vi "Thermal Chamber Response Simulator_Init-setup.vi"(11 "test case ID":string) -> (3 "Test Error":errorcluster)   [LabVIEW 2018]
doc: "The setup VI should be executed before the VI under test in the harness VI. In this VI you can prepare the environment and the inputs of the VI under test.\n\nSee the Help Document for more information. (<b>Help</b> > <b>IncQuery Labs</b> > <b>InstaCoverage</b> > <b>InstaCoverage Help...</b>)"
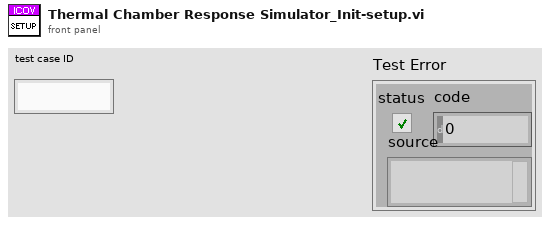
[diagram p1: front panel]
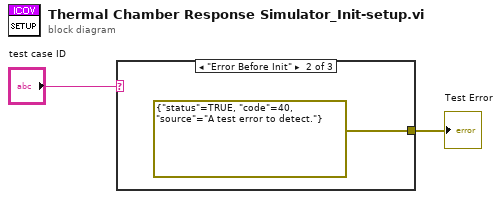
[diagram p0: block diagram]
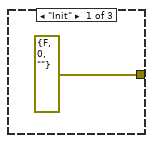
[diagram p2: hidden frame]
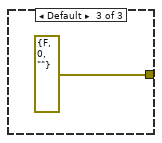
[diagram p3: hidden frame]
diagram:
  n1 = case shown="\"Error Before Init\"" "test case ID" {
    tunnel: [errorcluster {"status"=FALSE, "code"=0, "source"=""} ("error out") errorcluster {"status"=TRUE, "code"=40, "source"="A test error to detect."} ("error out") errorcluster {"status"=FALSE, "code"=0, "source"=""} ("error out")] -> w1
    frame "Init" {
    }
    frame "Error Before Init" {
    }
    frame Default {
    }
  }
  "Test Error" <- w1
